vi "UDP MCAST FGV.vi"(8 "error in":errorcluster, 10 "Function":enum16{"Read", "Write", "Clear"}(ring), 11 "UDP MCAST message in":string) -> (0 "error out":errorcluster, 3 "UDP MCAST message out":string)   [LabVIEW 2013, in "UDP_Mcast_Comm.lvlib"]
uses:
  UDP_Mcast_Comm.lvlib
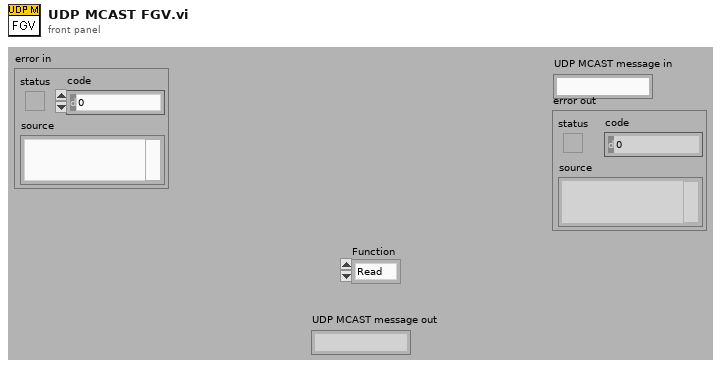
[diagram p1: front panel]
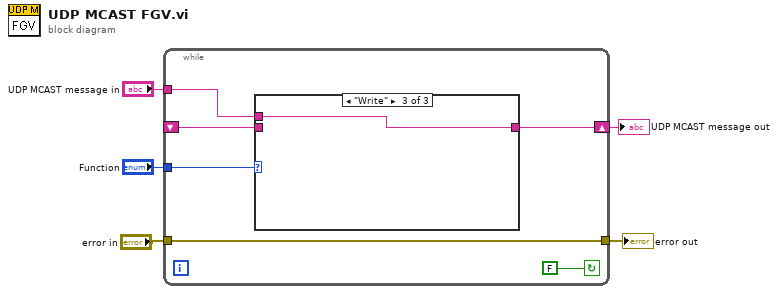
[diagram p0: block diagram]
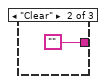
[diagram p3: hidden frame]
diagram:
  n1 = while {
    shift-right: [w9] -> w5
    shift-left: _ -> [w8]
    tunnel: "Function" -> [w11]
    tunnel: "UDP MCAST message in" -> [w10]
    tunnel: "error in" -> [w6]
    tunnel: [w6] -> w1
    stop <- FALSE continue-if-true
    n2 = case shown="\"Write\"" w11 {
      tunnel: w10 -> [_ _ w14]
      tunnel: [w12 "" w14] -> w9
      tunnel: w8 -> [w12 _ _]
      frame "Read", Default {
      }
      frame "Clear" {
      }
      frame "Write" {
      }
    }
  }
  "UDP MCAST message out" <- w5
  "error out" <- w1
